vi "detector_get_counts_1d_dbl.vi"(8 "error in (no error)":errorcluster, 11 "tt20 in":refnum<class "tt20.lvclass">) -> (0 "error out":errorcluster, 2 "counts":dbl[](array[numeric]), 3 "tt20 out":refnum<class "tt20.lvclass">)   [LabVIEW 2015, in "tt20.lvclass"]
uses:
  tt20.lvclass
  tt20.lvclass/tt20.ctl
  C:/Users/MX-Microscope/Documents/LabVIEW Data/lvoop_campus_2018/Detector_Class/Swabian/time_tagger_vis/TTCSharp32.dll
  time_tagger_vis/TTCSharp32.dll
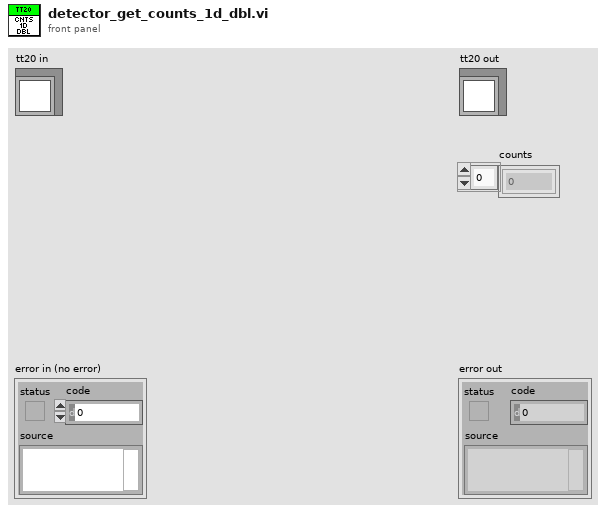
[diagram p1: front panel]
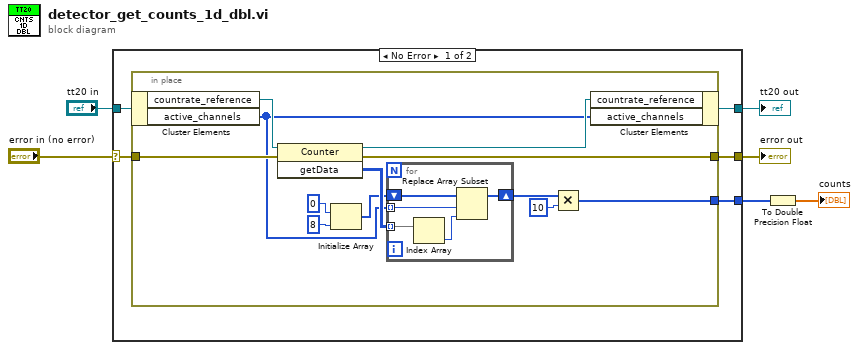
[diagram p0: block diagram]
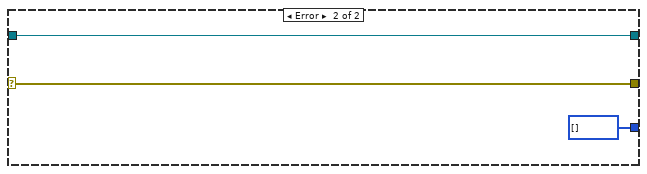
[diagram p2: hidden frame]
diagram:
  n1 = case shown="No Error" "error in (no error)" {
    selector: "error in (no error)" -> [w10 w31]
    tunnel: "tt20 in" -> [w11 w29]
    tunnel: [w9 w29] -> w4
    tunnel: [w7 i32[] [] ("getData")] -> w2
    tunnel: [w8 w31] -> w3
    frame No Error {
      n2 = in-place {
        in-place-border: w10 -> [w21]
        in-place-border: [w20] -> w8
        in-place-border: [w18] -> w7
        n3 = in-place-cluster #1(w11) -> ("countrate_reference"=w23:refnum<k24>, "active_channels"=w12:u32[])
        n4 = invoke class="Counter" method="getData"(reference=w23, error in=w21) -> (reference out=w22:refnum<k24>, error out=w20:errorcluster, "getData"=w17:i32[][])  [unwired: 1 in]
        n5 = Initialize Array(0, 8 ("dimension size")) -> (w14:i32[])
        n6 = for {
          tunnel: w17 -> [w28] mode=indexing
          tunnel: w12 -> [w27] mode=indexing
          shift-right: [w24] -> w13
          shift-left: w14 -> [w26]
          n7 = Index Array(array=w28) -> (element=w25:i32)  [unwired: 1 in]
          n8 = Replace Array Subset(array=w26, new element=w25, index=w27) -> (w24:i32[])
        }
        n9 = Multiply(x=w13, y=10) -> (x*y=w18:i32[])
        n10 = in-place-cluster #1("countrate_reference"=w22, "active_channels"=w12) -> (w9:refnum<class "tt20.lvclass">)
      }
    }
    frame Error {
    }
  }
  "error out" <- w3
  "tt20 out" <- w4
  n11 = To Double Precision Float(number=w2) -> (double precision float=→"counts":dbl[])
